vi "Parse Alarms Array.vi"(10 "alarms":T1[](array[typedef])=[{"alarm URL"="\\\\LASERBAY-DEV\\Logger Master\\LB_Amp1_Energy.Alarms.LB_Amp1_Energy", "set time"=timestamp(3511959737.5175076 s since 1904-01-01), "set user"="(Nobody)", "ack time"=timestamp(-9223372036854775808 s since 1904-01-01), "ack user"="", "clear time"=timestamp(-9223372036854775808 s since 1904-01-01), "clear user"="", "setpoint"=1200.0, "value"=1409.99, "priority"=1, "alarm area"="Laser Bay", "alarm description"="LB_Amp1_Energy", "ack comment"="", "event?"=FALSE, "Refnum"=216172782113783839}] {"value" format="%.2f"; "setpoint" format="%.2f"; "clear time" format="%<%X\n%x>T"; "ack time" format="%<%X\n%x>T"; "set time" format="%<%X\n%x>T"}, 11 "Alarms for Expt":string[](array[string])) -> (3 "Alarms Info":string[][](array[string]))   [LabVIEW 2018]
uses:
  Alarms--Cluster.ctl
panel:
  out "Numeric":i32
  out "Description":string[](array[string])
  out "Date/Time":string[](array[string])
  out "Set Point":string[](array[string])
  out "Value":string[](array[string])
  out "Variable Name":string[](array[string])
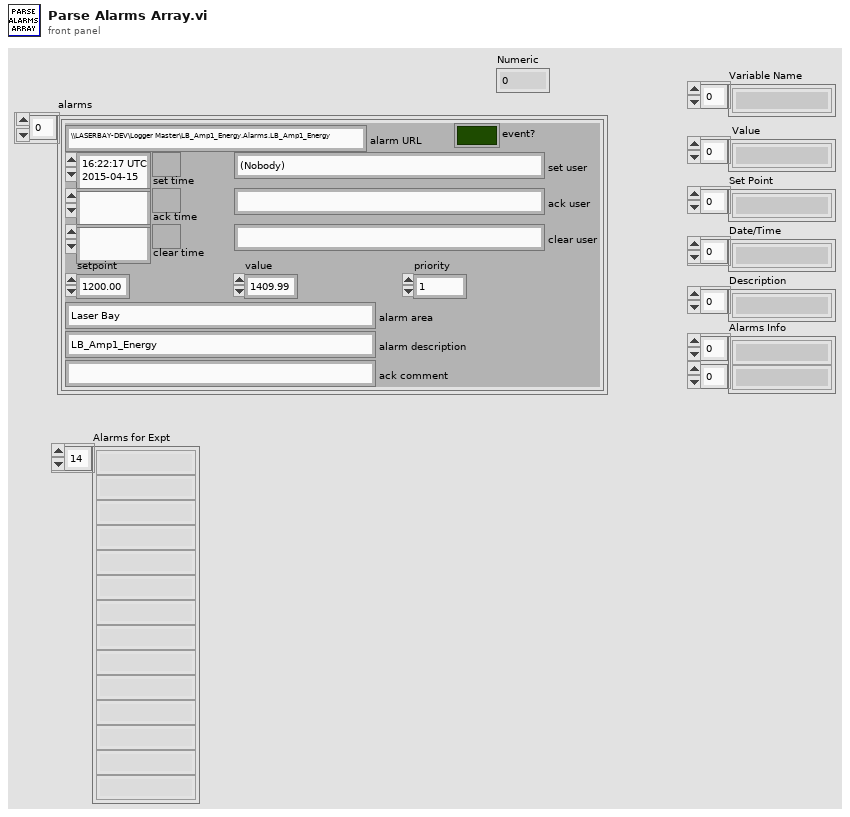
[diagram p1: front panel]
types:
  T1 = typedef "Alarms--Cluster.ctl" = cluster{"alarm URL":string, "set time":timestamp, "set user":string, "ack time":timestamp, "ack user":string, "clear time":timestamp, "clear user":string, "setpoint":dbl, "value":dbl, "priority":u32, "alarm area":string, "alarm description":string, "ack comment":string, "event?":bool, "Refnum":u64}
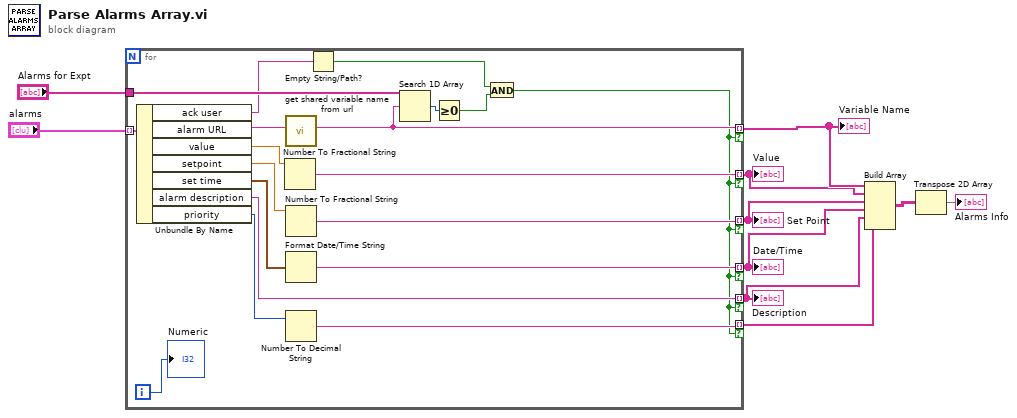
[diagram p0: block diagram]
diagram:
  n1 = for {
    tunnel: "alarms" -> [w29] mode=indexing
    tunnel: [w16] -> w9 mode=indexing if=w11
    tunnel: [w26] -> w8 mode=indexing if=w11
    tunnel: [w24] -> w7 mode=indexing if=w11
    tunnel: [w22] -> w6 mode=indexing if=w11
    tunnel: [w21] -> w5 mode=indexing if=w11
    tunnel: [w19] -> w2 mode=indexing if=w11
    tunnel: "Alarms for Expt" -> [w17]
    i -> [w18]
    n2 = Unbundle By Name(w29) -> ("ack user"=w14:string, "alarm URL"=w28:string, "value"=w27:dbl, "setpoint"=w25:dbl, "set time"=w23:timestamp, "alarm description"=w21:string, "priority"=w20:u32)
    n3 = Number To Fractional String(number=w27) -> (F-format string=w26:string)  [unwired: 3 in]
    n4 = call "get shared variable name from url.vi"("string in"=w28) -> ("Shared Variable"=w16:string)  [unwired: 9 in, 1 out]
    n5 = Number To Fractional String(number=w25) -> (F-format string=w24:string)  [unwired: 3 in]
    n6 = Format Date/Time String(seconds (now)=w23) -> (date/time string=w22:string)  [unwired: 2 in]
    n7 = Number To Decimal String(number=w20) -> (decimal integer string=w19:string)  [unwired: 1 in]
    n8 = Empty String/Path?(string/path=w14) -> (empty?=w12:bool)
    n9 = Search 1D Array(1D array=w17, element=w16) -> (index of element=w15:i32)  [unwired: 1 in]
    n10 = Greater Or Equal To 0?(x=w15) -> (x >= 0?=w13:bool)
    n11 = And(x=w12, y=w13) -> (x .and. y?=w11:bool)
    "Numeric" <- w18
  }
  "Variable Name" <- w9
  "Value" <- w8
  "Set Point" <- w7
  "Date/Time" <- w6
  "Description" <- w5
  n12 = Build Array(w9, w8, w7, w6, w5, w2) -> (w4:string[][])
  n13 = Transpose 2D Array(2D array=w4) -> (transposed array=→"Alarms Info":string[][])
